vi "SIAM-ScaleDirekt.vi"(7 "ScaleConst":T1(array[cluster])=[{"Axis-Ring"=104857665, "Scale"=-128000.0, "Offset"=-1000000.0, "HW min"=-3000000.0, "HW max"=0.0, "max a"=inf, "units"="µm"}, {"Axis-Ring"=102760513, "Scale"=65536.0, "Offset"=-4000.0, "HW min"=0.0, "HW max"=inf, "max a"=inf, "units"="c"}, {"Axis-Ring"=101711937, "Scale"=65536.0, "Offset"=0.0, "HW min"=0.0, "HW max"=inf, "max a"=inf, "units"="c"}, {"Axis-Ring"=16777217, "Scale"=51200.0, "Offset"=100.0, "HW min"=0.0, "HW max"=5500000.0, "max a"=inf, "units"="mm"}, {"Axis-Ring"=17825793, "Scale"=51200.0, "Offset"=100.0, "HW min"=0.0, "HW max"=3700000.0, "max a"=inf, "units"="mm"}, {"Axis-Ring"=19922945, "Scale"=153600.0, "Offset"=146600.0, "HW min"=0.0, "HW max"=614400.0, "max a"=inf, "units"="Pos"}, {"Axis-Ring"=20971521, "Scale"=25000.1, "Offset"=641.0, "HW min"=0.0, "HW max"=124721.0, "max a"=inf, "units"="Pos"}, {"Axis-Ring"=22020097, "Scale"=1.0, "Offset"=0.0, "HW min"=0.0, "HW max"=51200.0, "max a"=inf, "units"="counts"}, {"Axis-Ring"=23068673, "Scale"=10240.0, "Offset"=0.0, "HW min"=0.0, "HW max"=51200.0, "max a"=inf, "units"="Pos"}, {"Axis-Ring"=24117249, "Scale"=1.0, "Offset"=0.0, "HW min"=0.0, "HW max"=51200.0, "max a"=inf, "units"="counts"}, {"Axis-Ring"=2684354561, "Scale"=1.0, "Offset"=0.0, "HW min"=0.0, "HW max"=65636.0, "max a"=inf, "units"="counts"}, {"Axis-Ring"=2685403137, "Scale"=1.0, "Offset"=0.0, "HW min"=0.0, "HW max"=65636.0, "max a"=inf, "units"="counts"}, {"Axis-Ring"=2686451713, "Scale"=1.0, "Offset"=0.0, "HW min"=0.0, "HW max"=65636.0, "max a"=inf, "units"="counts"}, {"Axis-Ring"=2687500289, "Scale"=1.0, "Offset"=0.0, "HW min"=0.0, "HW max"=65636.0, "max a"=inf, "units"="counts"}, {"Axis-Ring"=2688548865, "Scale"=1.0, "Offset"=0.0, "HW min"=0.0, "HW max"=65636.0, "max a"=inf, "units"="counts"}, {"Axis-Ring"=2689597441, "Scale"=1.0, "Offset"=1.0, "HW min"=0.0, "HW max"=65636.0, "max a"=inf, "units"="counts"}, {"Axis-Ring"=2690646017, "Scale"=1.0, "Offset"=1.0, "HW min"=0.0, "HW max"=65636.0, "max a"=inf, "units"="counts"}, {"Axis-Ring"=2691694593, "Scale"=1.0, "Offset"=1.0, "HW min"=0.0, "HW max"=65636.0, "max a"=inf, "units"="counts"}, {"Axis-Ring"=2701131777, "Scale"=1.0, "Offset"=1.0, "HW min"=0.0, "HW max"=65636.0, "max a"=inf, "units"="counts"}, {"Axis-Ring"=2702180353, "Scale"=1.0, "Offset"=1.0, "HW min"=0.0, "HW max"=65636.0, "max a"=inf, "units"="counts"}, {"Axis-Ring"=2703228929, "Scale"=1.0, "Offset"=1.0, "HW min"=0.0, "HW max"=65636.0, "max a"=inf, "units"="counts"}, {"Axis-Ring"=2704277505, "Scale"=1.0, "Offset"=1.0, "HW min"=0.0, "HW max"=65636.0, "max a"=inf, "units"="counts"}, {"Axis-Ring"=2717908993, "Scale"=1.0, "Offset"=1.0, "HW min"=0.0, "HW max"=65636.0, "max a"=inf, "units"="counts"}, {"Axis-Ring"=2718957569, "Scale"=1.0, "Offset"=1.0, "HW min"=0.0, "HW max"=65636.0, "max a"=inf, "units"="counts"}, {"Axis-Ring"=2720006145, "Scale"=1.0, "Offset"=1.0, "HW min"=0.0, "HW max"=65636.0, "max a"=inf, "units"="counts"}, {"Axis-Ring"=2721054721, "Scale"=1.0, "Offset"=1.0, "HW min"=0.0, "HW max"=65636.0, "max a"=inf, "units"="counts"}, {"Axis-Ring"=67108865, "Scale"=1.0, "Offset"=1.0, "HW min"=100000.0, "HW max"=200000.0, "max a"=inf, "units"="counts"}, {"Axis-Ring"=68157441, "Scale"=1.0, "Offset"=1.0, "HW min"=100000.0, "HW max"=200000.0, "max a"=inf, "units"="counts"}] {"Axis-Ring" items=["Galvo1"=101711937, "x-Galvo"=102760513, "z-Fokus"=104857665, "X-Axis"=16777217, "Y-Axis"=17825793, "Obj"=19922945, "Filter"=20971521, "Trans"=22020097, "FRET"=23068673, "SI"=24117249, "LED385"=2685403137, "LED440"=2686451713, "LED470"=2687500289, "LED510"=2688548865, "LED540"=2689597441, "LED590"=2690646017, "LED640"=2691694593, "DurchR"=2701131777, "DurchG"=2702180353, "DurchB"=2703228929, "AF"=2704277505, "Laser0"=2717908993, "Laser1"=2718957569, "Laser2"=2720006145, "Laser3"=2721054721, "Servo0"=67108865, "Servo1"=68157441]}, 11 "Linear":cluster{"Axis-Ring":u32, "Position":i32}={"Axis-Ring"=16777217, "Position"=506438} {"Axis-Ring" items=["X-Axis"=16777217, "Y-Axis"=17825793, "Obj"=19922945, "Filter"=20971521, "Trans"=22020097, "FRET"=23068673, "SI"=24117249, "LED365"=2684354561, "LED385"=2685403137, "LED440"=2686451713, "LED470"=2687500289, "LED510"=2688548865, "LED540"=2689597441, "LED590"=2690646017, "LED640"=2691694593, "DurchR"=2701131777, "DurchG"=2702180353, "DurchB"=2703228929, "AF"=2704277505, "Laser0"=2717908993, "Laser1"=2718957569, "Laser2"=2720006145, "Laser3"=2721054721, "Servo0"=67108865, "Servo1"=68157441]; "Position" scale=0.0..250.0}) -> (3 "Array":T3(array[cluster]) {"Device" format="%x" items=["read_x-Motor_status_ticket"=17305600, "init_x-Motor"=17760263, "read_x-Motor_absolute_ticket"=16781312, "move_x-Motor_absolute"=16777217, "move_x-Motor_relative"=16842753, "read_x-Motor_speed"=16977920, "set_x-Motor_speed"=16973825, "read_y-Motor_status_ticket"=18354176, "init_y-Motor"=18808839, "read_y-Motor_absolute_ticket"=17829888, "move_y-Motor_absolute"=17825793, "move_y-Motor_relative"=17891329, "read_y-Motor_speed"=18026496, "set_y-Motor_speed"=18022401, "read_z-Motor_status_ticket"=19402752, "init_z-Motor"=19857415, "stop_z-Motor"=19857423, "start_z-Motor"=19857422, "read_z-Motor_absolute_ticket"=18878464, "move_z-Motor_absolute"=18874369, "move_z-Motor_relative"=18939905, "read_Objective_status_ticket"=20451328, "init_Objective"=20905991, "read_Objective_absolute_ticket"=19927040, "move_Objective_absolute"=19922945, "move_Objective_relative"=19988481, "read_Objective-Motor_speed"=20123648, "set_Objective-Motor_speed"=20119553, "read_Filter_status_ticket"=21499904, "init_Filter"=21954567, "read_Filter_absolute_ticket"=20975616, "move_Filter_absolute"=20971521, "move_Filter_relative"=21037057, "read_Filter-Motor_speed"=21172224, "set_Filter-Motor_speed"=21168129, "read_Trans-Rad_status_ticket"=22548480, "init_Trans-Rad"=23003143, "read_Trans-Rad_absolute_ticket"=22024192, "move_Trans-Rad_absolute"=22020097, "move_Trans-Rad_relative"=22085633, "read_Trans-Motor_speed"=22220800, "set_Trans-Motor_speed"=22216705, "read_FRET_status_ticket"=23597056, "init_FRET"=24051719, "read_FRET_absolute_ticket"=23072768, "move_FRET_absolute"=23068673, "move_FRET_relative"=23134209, "read_FRET-Motor_speed"=23269376, "set_FRET-Motor_speed"=23265281, "read_SI-Rad_status_ticket"=24645632, "init_SI-Rad"=25100295, "read_SI-Rad_absolute_ticket"=24121344, "move_SI-Rad_absolute"=24117249, "move_SI-Rad_relative"=24182785, "read_SI-Rad_speed"=24317952, "set_SI-Rad_speed"=24313857, "I2C-write"=335544321, "I2C-read"=335548416, "end_no_ticket"=4027514895, "end_ticket"=4027518991, "IO-read_bank0"=3489665024, "IO-write_bank0"=3489660929, "IO-read_bank1"=3506442240, "IO-write_bank1"=3506438145, "DA0-0_LED365"=2684354561, "DA0-1_LED385"=2685403137, "DA0-2_LED440"=2686451713, "DA0-3_LED470"=2687500289, "DA0-4_LED510"=2688548865, "DA0-5_LED550"=2689597441, "DA0-6_LED590"=2690646017, "DA0-7_LED640"=2691694593, "DA1-0_LED-R"=2701131777, "DA1-1_LED-G"=2702180353, "DA1-2_LED-B"=2703228929, "DA1-3_LED-AF"=2704277505, "DA1-4"=2705326081, "DA1-5"=2706374657, "DA1-6"=2707423233, "DA1-7"=2708471809, "DA2-Laser0"=2717908993, "DA2-Laser1"=2718957569, "DA2-Laser2"=2720006145, "DA2-Laser3"=2721054721, "DA2-Laser4"=2722103297, "Analog-read_AD0-0"=2818576384, "Analog-read-store_AD0-0"=2818572290, "IO-delay_bank0"=3489923073, "IO-delay_bank0_fromVar"=3489923075, "read_cam_clock"=3289124864, "store_cam_clock"=3289120770, "read_cam_phase"=3289190400, "store_cam_phase"=3289190402, "Read ticks"=4027518976, "Read ticks to var"=4027518978, "Read IP"=4043313152, "Read IP into var"=4043313154, "Set IP from var"=4043309059, "Set IP from var, relative"=4043313155, "decrement_branchRel_if_equal"=4043374945, "decrement_branchRel_if_greaterequal"=4043375201, "decrement_branchRel_if_greaterequal_withTicket"=4043379297, "decrement_branchRel_if_smaller"=4043375457, "increment_branchRel_if_smaller"=4043375473, "readVar"=4060090368, "writeVar"=4060086273, "readVar_and_copy_to_var2"=4060086275, "loadVar2_andcopy_var1"=4060086276, "math_addToVariable"=4076863488, "math_addVToVariable"=4076863489, "math_subToVariable"=4076863490, "math_subVToVariable"=4076863491, "math_multToVariable"=4076863492, "math_multvToVariable"=4076863493, "math_divideToVariable"=4076863494, "math_divideVToVariable"=4076863495, "math_modToVariable"=4076863496, "math_modVToVariable"=4076863497, "logic_and"=4093640704, "logic_or"=4093640706, "logic_xor"=4093640708, "set_1Galvo"=101712113, "set_x-Galvo"=102760689, "set_y-Galvo"=103809265, "set_z-Fokus"=104857841, "set_1Galvo_position-only"=101711937, "set_x-Galvo_position-only"=102760513, "set_y-Galvo_position-only"=103809089, "set_z-Fokus_position-only"=104857665, "set_x-Galvo_position-only_ticket"=102764609, "set_y-Galvo_position-only_ticket"=103813185, "set_z-Fokus_position-only_ticket"=104861761, "set_x-Galvo_relativ-only"=102760577, "set_y-Galvo_relativ-only"=103809153, "set_z-Fokus_relativ-only"=104857729, "set_x-Galvo_speed-only"=102760481, "set_y-Galvo_speed-only"=103809057, "set_z-Fokus_speed-only"=104857633, "read_1Galvo_ticket"=101716032, "read_x-Galvo_ticket"=102764608, "read_y-Galvo_ticket"=103813184, "read_z-Focus_ticket"=104861760, "x-Galvo_pos_fromVar"=102760515, "y-Galvo_pos_fromVar"=103809091, "z-Focus_pos_fromVar"=104857667, "Servo0"=67108865, "Servo0-enable"=68091911, "Servo0-disable"=68091919, "Servo1"=68157441, "Servo1-enable"=69140487, "Servo1-disable"=69140495, "EnablePower0-SM"=2148466695, "DisablePower0-SM"=2148466703, "EnablePower1-Thermo1"=2149515271, "DisablePower1-Thermo1"=2149515279, "EnablePower2-Cam"=2150563847, "DisablePower2-Cam"=2150563855, "EnablePower3-Thermo2"=2151612423, "DisablePower3-Thermo2"=2151612431, "EnablePower4-Laser0"=2152660999, "DisablePower4-Laser0"=2152661007, "EnablePower5"=2153709575, "DisablePower5"=2153709583, "EnablePower6-Laser1"=2154758151, "DisablePower6-Laser1"=2154758159, "EnablePower7-SAM"=2155806727, "DisablePower7-SAM"=2155806735, "EnablePower8-Laser2"=2156855303, "DisablePower8-Laser2"=2156855311, "EnablePower9-TSM"=2157903879, "DisablePower9-TSM"=2157903887, "EnablePower10-Laser3"=2158952455, "DisablePower10-Laser3"=2158952463, "EnablePower11-Servo"=2160001031, "DisablePower11-Servo"=2160001039, "EnablePower12-Laser4"=2161049607, "DisablePower12-Laser4"=2161049615, "EnableSMPower2-DCC22"=2167341063, "DisableSMPower2-DCC22"=2167341071, "EnableSMPower3-6220"=2168389639, "DisableSMPower3-6220"=2168389647, "EnableSMPower4-6210"=2169438215, "DisableSMPower4-6210"=2169438223]})   [LabVIEW 2011]
uses:
  SIAM_command.ctl
panel:
  out "In Range?":bool
  out "x+y":dbl
  out "number":dbl
  out "Scaled":bool
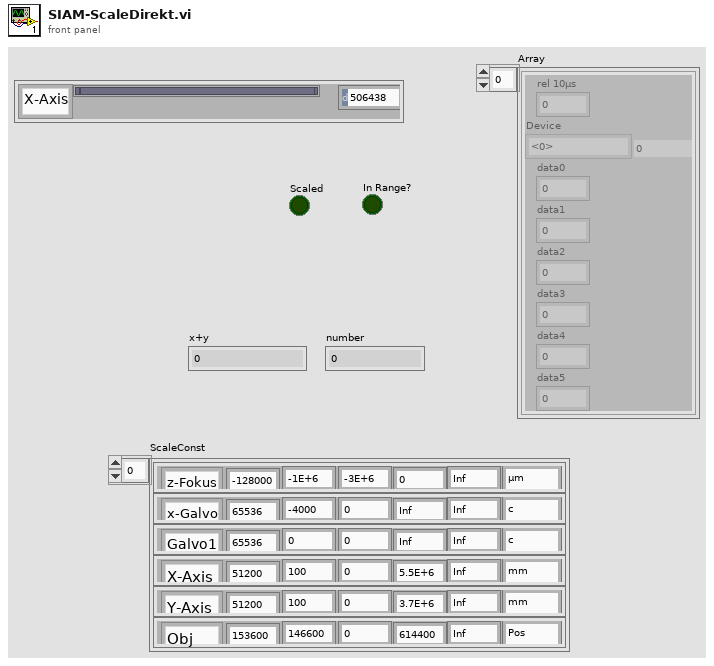
[diagram p1: front panel]
types:
  T1 = cluster{"Axis-Ring":u32, "Scale":dbl, "Offset":dbl, "HW min":dbl, "HW max":dbl, "max a":dbl, "units":string}[]
  T2 = typedef "SIAM_command.ctl" = u32
  T3 = cluster{"rel 10µs":u32, "Device":T2, "data0":i32, "data1":i32, "data2":i32, "data3":i32, "data4":i32, "data5":i32}[]
  T4 = cluster{"rel 10µs":u32, "Device":T2, "data0":i32, "data1":i32, "data2":i32, "data3":i32, "data4":i32, "data5":i32}
  T5 = cluster{"Axis-Ring":u32, "Scale":dbl, "Offset":dbl, "HW min":dbl, "HW max":dbl, "max a":dbl, "units":string}
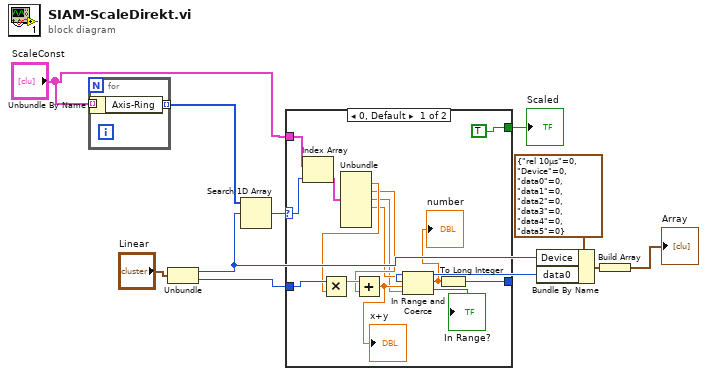
[diagram p0: block diagram]
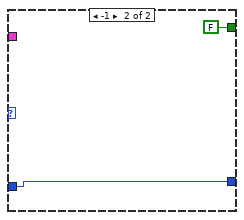
[diagram p2: hidden frame]
diagram:
  n1 = for {
    tunnel: "ScaleConst" -> [w13] mode=indexing
    tunnel: [w12] -> w3 mode=indexing
    n2 = Unbundle By Name(w13) -> ("Axis-Ring"=w12:u32)
  }
  n3 = Unbundle("Linear") -> ("Axis-Ring"=w7:u32, "Position"=w5:i32)
  n4 = Search 1D Array(1D array=w3, element=w7) -> (index of element=w6:i32)  [unwired: 1 in]
  n5 = case shown="0, Default" w6 {
    selector: w6 -> [w25 _]
    tunnel: w5 -> [w27 w29]
    tunnel: [w19 w29] -> w4
    tunnel: "ScaleConst" -> [w26 _]
    tunnel: [TRUE FALSE] -> w1
    frame 0, Default {
      n6 = Index Array(array=w26, index=w25) -> (element=w24:T5)
      n7 = Unbundle(w24) -> ("Scale"=w21:dbl, "Offset"=w20:dbl, "HW min"=w14:dbl, "HW max"=w15:dbl)  [unwired: 3 out]
      n8 = Multiply(x=w27, y=w21) -> (x*y=w23:dbl)
      n9 = Add(x=w23, y=w20) -> (x+y=w22:dbl)
      "x+y" <- w22
      n10 = In Range and Coerce(upper limit=w15, x=w22, lower limit=w14) -> (coerced(x)=w17:dbl, In Range?=→"In Range?":bool)
      "number" <- w17
      n11 = To Long Integer(number=w17) -> (32bit integer=w19:i32)
    }
    frame -1 {
    }
  }
  "Scaled" <- w1
  n12 = Bundle By Name(cluster=T4 {"rel 10µs"=0, "Device"=0, "data0"=0, "data1"=0, "data2"=0, "data3"=0, "data4"=0, "data5"=0} ("output cluster"), "Device"=w7, "data0"=w4) -> (w8:T4)
  n13 = Build Array(w8) -> (→"Array":T3)
